vi "Read Device 2.vi"(8 "error in (no error)":errorcluster, 11 "AlicatPressureController in":refnum<class "AlicatPressureController.lvclass">) -> (0 "error out":errorcluster, 3 "AlicatPressureController out":refnum<class "AlicatPressureController.lvclass">)   [LabVIEW 2020, in "AlicatPressureController.lvclass"]
uses:
  AlicatPressureController.lvclass
  AlicatPressureController.lvclass/AlicatPressureController.ctl
  OnOffTypeDef.ctl
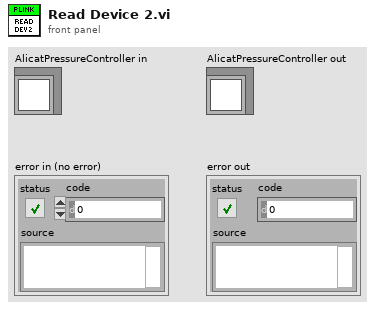
[diagram p1: front panel]
types:
  T1 = typedef "OnOffTypeDef.ctl" = enum16{"off", "on"}
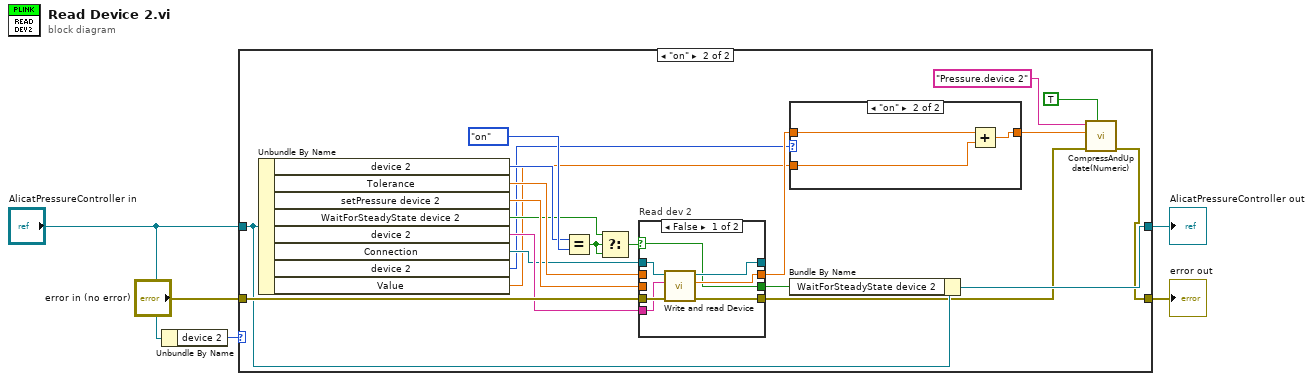
[diagram p0: block diagram]
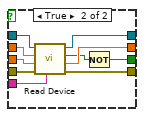
[diagram p4: hidden frame]
diagram:
  n1 = Unbundle By Name("AlicatPressureController in") -> ("device 2"=w2:T1)
  n2 = case shown="\"on\"" w2 {
    tunnel: "error in (no error)" -> [w7 w28]
    tunnel: [w7 w8] -> w3
    tunnel: "AlicatPressureController in" -> [w6 w14]
    tunnel: [w6 w13] -> w5
    frame "off", Default {
    }
    frame "on" {
      n3 = Unbundle By Name(w14) -> ("device 2"=w24:T1, "Tolerance"=w23:dbl, "setPressure device 2"=w22:dbl, "WaitForSteadyState device 2"=w21:bool, "device 2"=w20:string, "Connection"=w19:refnum<visa-resource-name>, "device 2"=w17:T1, "Value"=w16:dbl)
      n4 = Equal?(x=w24, y=OnOffTypeDef."on") -> (x = y?=w26:bool)
      n5 = Select(t=w21, s=w26, f=w26) -> (s? t:f=w25:bool)
      n6 = case "Read dev 2" shown="False" w25 {
        selector: w25 -> [w33 _]
        tunnel: w28 -> [w39 w49]
        tunnel: [w35 w48] -> w9
        tunnel: [w36 w47] -> _
        tunnel: [w34 w46] -> w18
        tunnel: w19 -> [w37 w45]
        tunnel: w20 -> [w38 w41]
        tunnel: w22 -> [_ w43]
        tunnel: w23 -> [_ w44]
        tunnel: [w33 w40] -> w15
        frame False {
          n7 = call "Write and read Device.vi"("error in (no error)"=w39, "device 1"=w38, "VISA Refnum in"=w37) -> ("error out"=w35:errorcluster, "pressure reading"=w34:dbl, "VISA Refnum out"=w36:refnum<visa-resource-name>)  [unwired: 5 in, 1 out]
        }
        frame True {
          n8 = call "Read Device.vi"("device address"=w41, "error in (no error)"=w49, "setPressure"=w43, "Tolerance"=w44, "VISA Refnum in"=w45) -> ("error out"=w48:errorcluster, ">Reading in native controller units>"=w46:dbl, "Boolean"=w42:bool, "VISA Refnum out"=w47:refnum<visa-resource-name>)  [unwired: 3 in]
          n9 = Not(x=w42) -> (.not. x?=w40:bool)
        }
      }
      n10 = case shown="\"on\"" w17 {
        tunnel: w18 -> [w29 w32]
        tunnel: [w29 w31] -> w10
        tunnel: w16 -> [_ w30]
        frame "off", Default {
        }
        frame "on" {
          n11 = Add(x=w32, y=w30) -> (x+y=w31:dbl)
        }
      }
      n12 = Bundle By Name(cluster=w14, "WaitForSteadyState device 2"=w15) -> (w13:refnum<class "AlicatPressureController.lvclass">)
      n13 = call "CompressAndUpdate(Numeric).vi"("force CVT update (false)"=TRUE, "error in"=w9, "Numeric"=w10, "command or variable name"="Pressure.device 2") -> ("error out"=w8:errorcluster)  [unwired: 7 in]
    }
  }
  "AlicatPressureController out" <- w5
  "error out" <- w3
